vi "PQcancel.vi"(8 "error in (no error)":errorcluster, 9 "errbufsize":i32=256, 10 "errbuf":string, 11 "cancel":u32) -> (0 "error out":errorcluster, 1 "PQcancel":i32, 2 "errbuf out":string, 3 "cancel_out":u32)   [LabVIEW 2019, in "libpqlv.lvlib"]
uses:
  libpqlv.lvlib
  libpq.dll
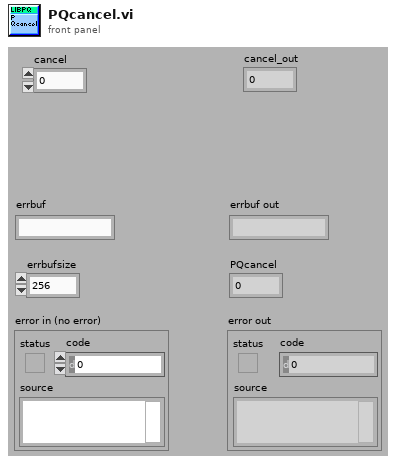
[diagram p1: front panel]
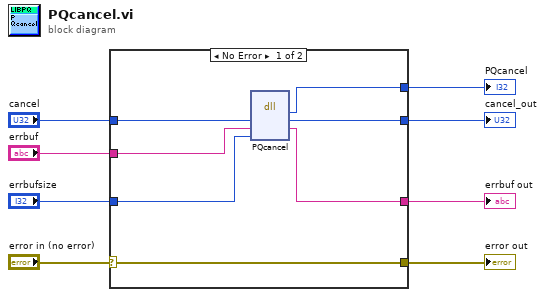
[diagram p0: block diagram]
diagram:
  n1 = case shown="No Error" "error in (no error)" {
    selector: "error in (no error)" -> [w15 w18]
    tunnel: [w15 w18] -> w7
    tunnel: [w14 _] -> w6
    tunnel: "errbuf" -> [w13 w17]
    tunnel: [w12 w17] -> w4
    tunnel: "errbufsize" -> [w11 _]
    tunnel: [w10 w16] -> w2
    tunnel: "cancel" -> [w9 w16]
    frame No Error {
      n2 = dll-call lib="libpq.*" fn="PQcancel"("cancel"=w9, "errbuf"=w13, "errbufsize"=w11) -> ("PQcancel"=w14:i32, "cancel"=w10:u32, "errbuf"=w12:string)  [unwired: 4 in, 2 out]
    }
    frame Error {
    }
  }
  "PQcancel" <- w6
  "errbuf out" <- w4
  "error out" <- w7
  "cancel_out" <- w2
